vi "VisualizeRTdataExternal.vi"(0 "ExitExternalPrograms":refnum<notifier>, 2 "path":path=path "C:/Users/olaja/Dropbox (Personal)/BME/IAF DATA/March30_2021/March_30_A", 4 "RTData/PPData":bool, 5 "error in (no error)":errorcluster) -> (19 "error out":errorcluster)   [LabVIEW 2021]
uses:
  <vilib>/Utility/file.llb/Read Delimited Spreadsheet (string).vi
  <vilib>/Utility/file.llb/Read Delimited Spreadsheet (DBL).vi
  <vilib>/Analysis/NI_AALBase.lvlib
panel:
  out "Current Experiment":string
  out "XY Graph":cluster{dbl[], dbl[]}[](graph)
  in  "Histogram intervals":i32=10
  in  "Xaxis":u16(ring) items=["Left", "Top", "Right", "Bottom", "Rotation", "CenterOfMassX", "CenterOfMassY", "FirstPixelY", "Area", "Mean Intensity", "Standard  Deviation", "Minimum Intensity", "Maximum Intensity", "FrameIndex"]
  in  "Yaxis":u16(ring) items=["Left", "Top", "Right", "Bottom", "Rotation", "CenterOfMassX", "CenterOfMassY", "FirstPixelY", "Area", "Mean Intensity", "Standard  Deviation", "Minimum Intensity", "Maximum Intensity", "FrameIndex"]
  out "Histogram Graph":T1(graph)
  in  "Refresh":bool
  # "If you want to visualize a new Experiment, Close this window and open it again from Main UI"
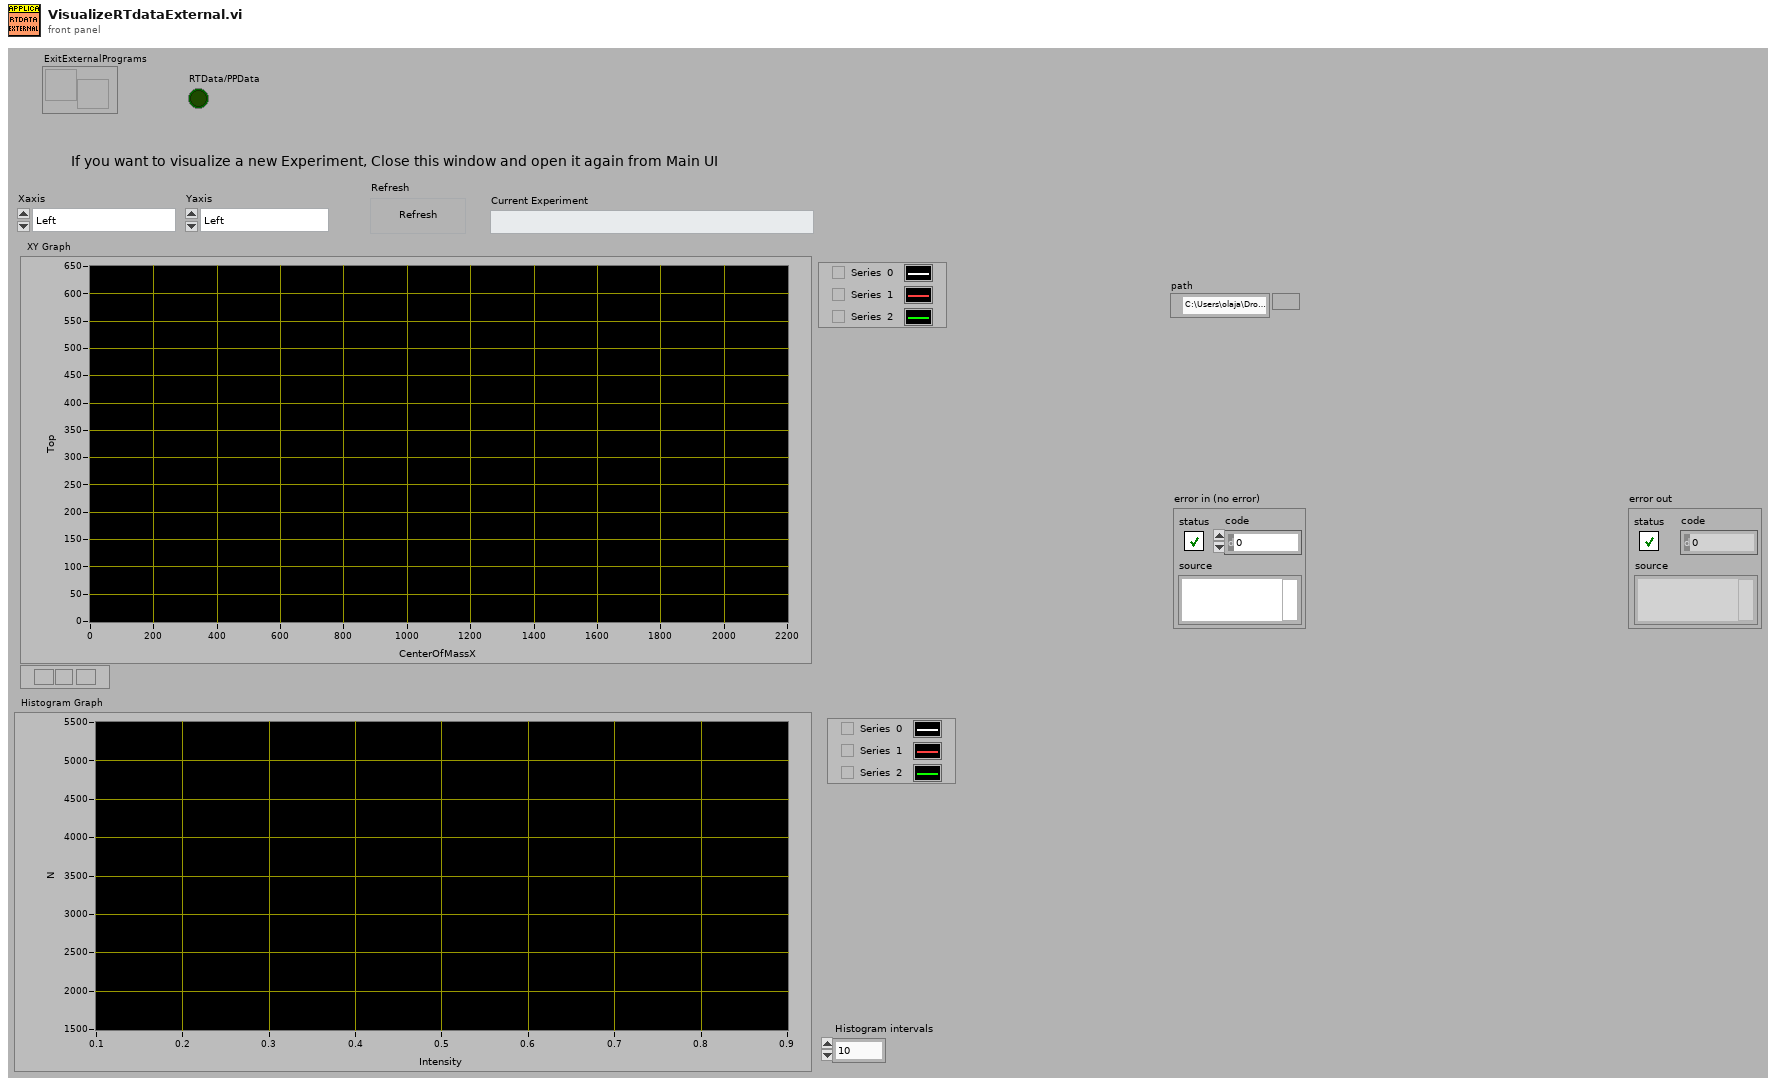
[diagram p1: front panel]
types:
  T1 = cluster{"X Values":dbl[], "Histogram: h(x)":i32[]}[]
  T2 = cluster{"X Values":dbl[], "Histogram: h(x)":i32[]}
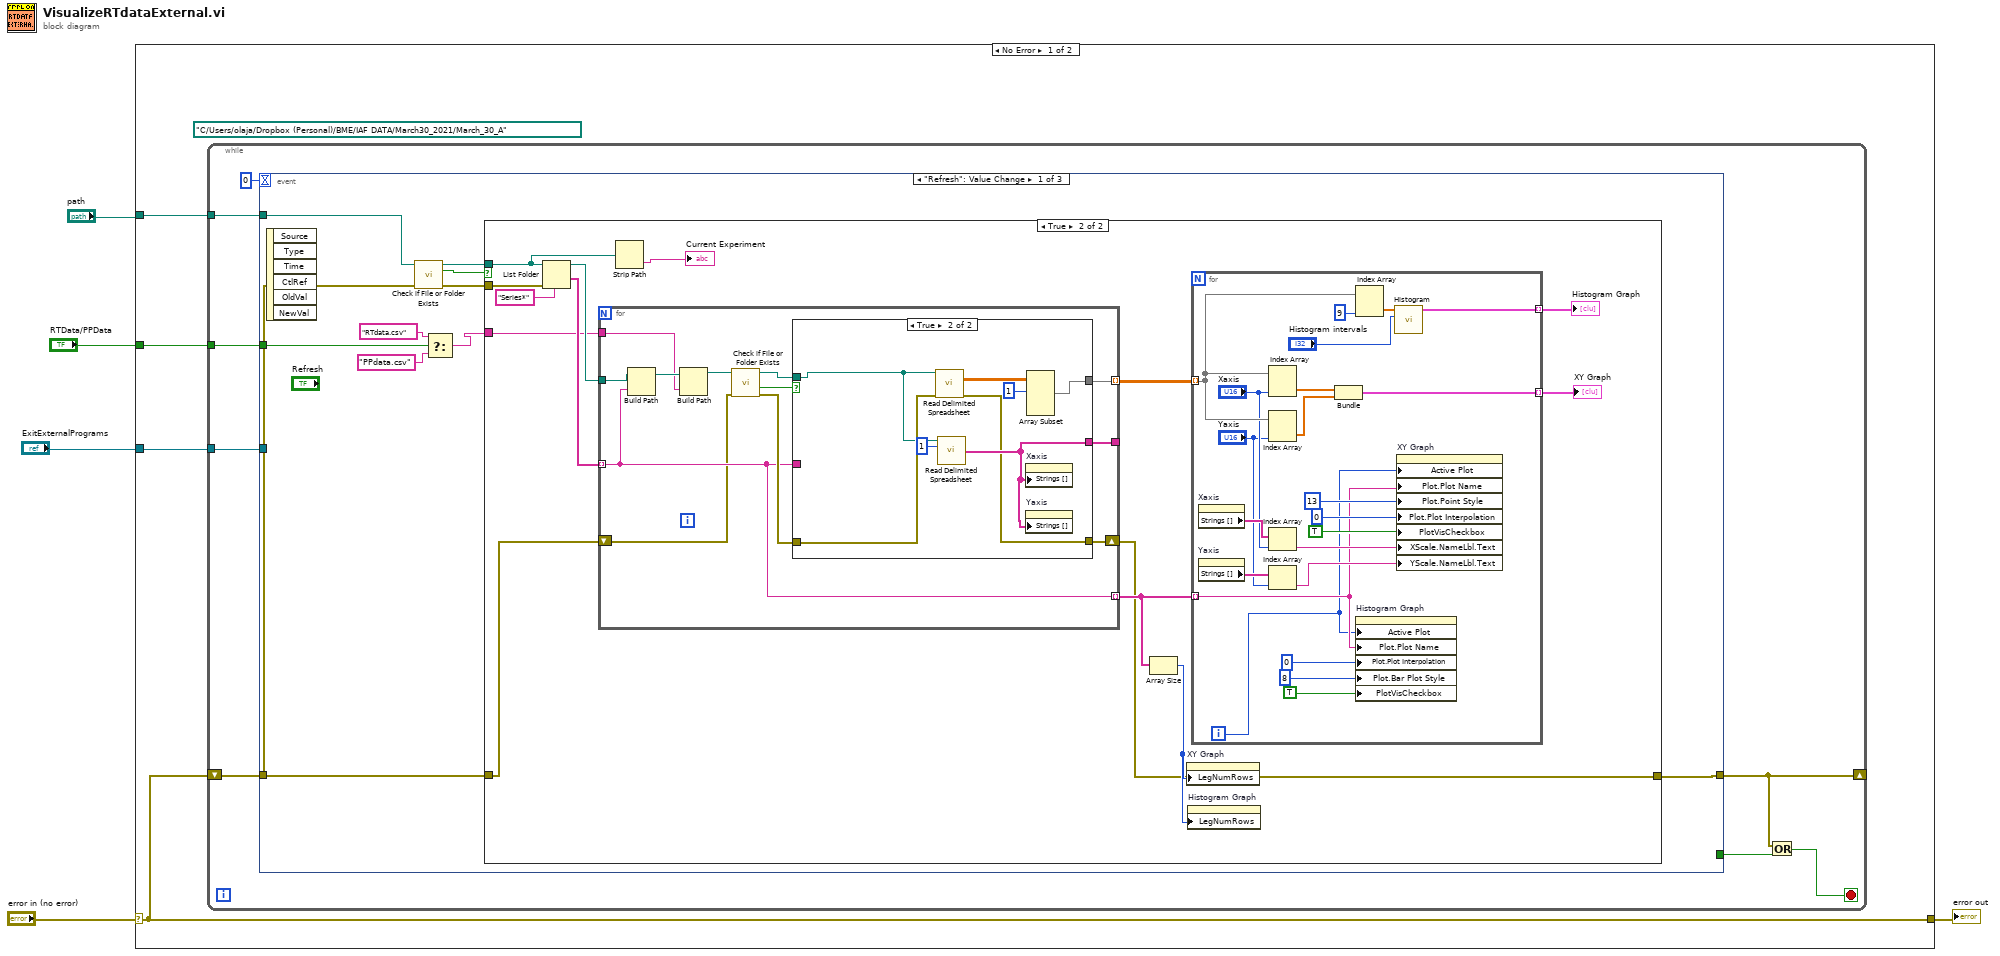
[diagram p0: block diagram]
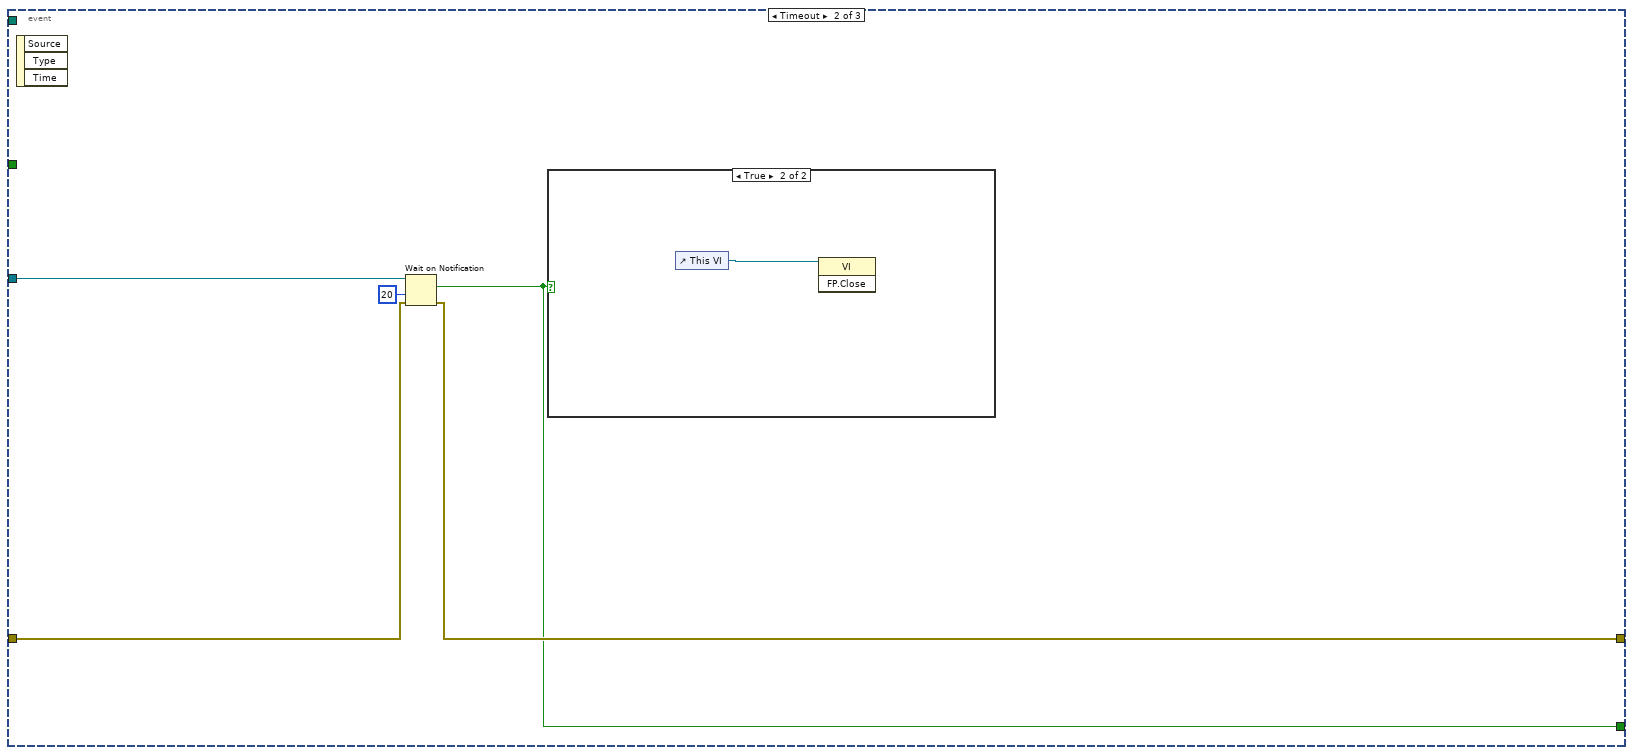
[diagram p4: hidden frame]
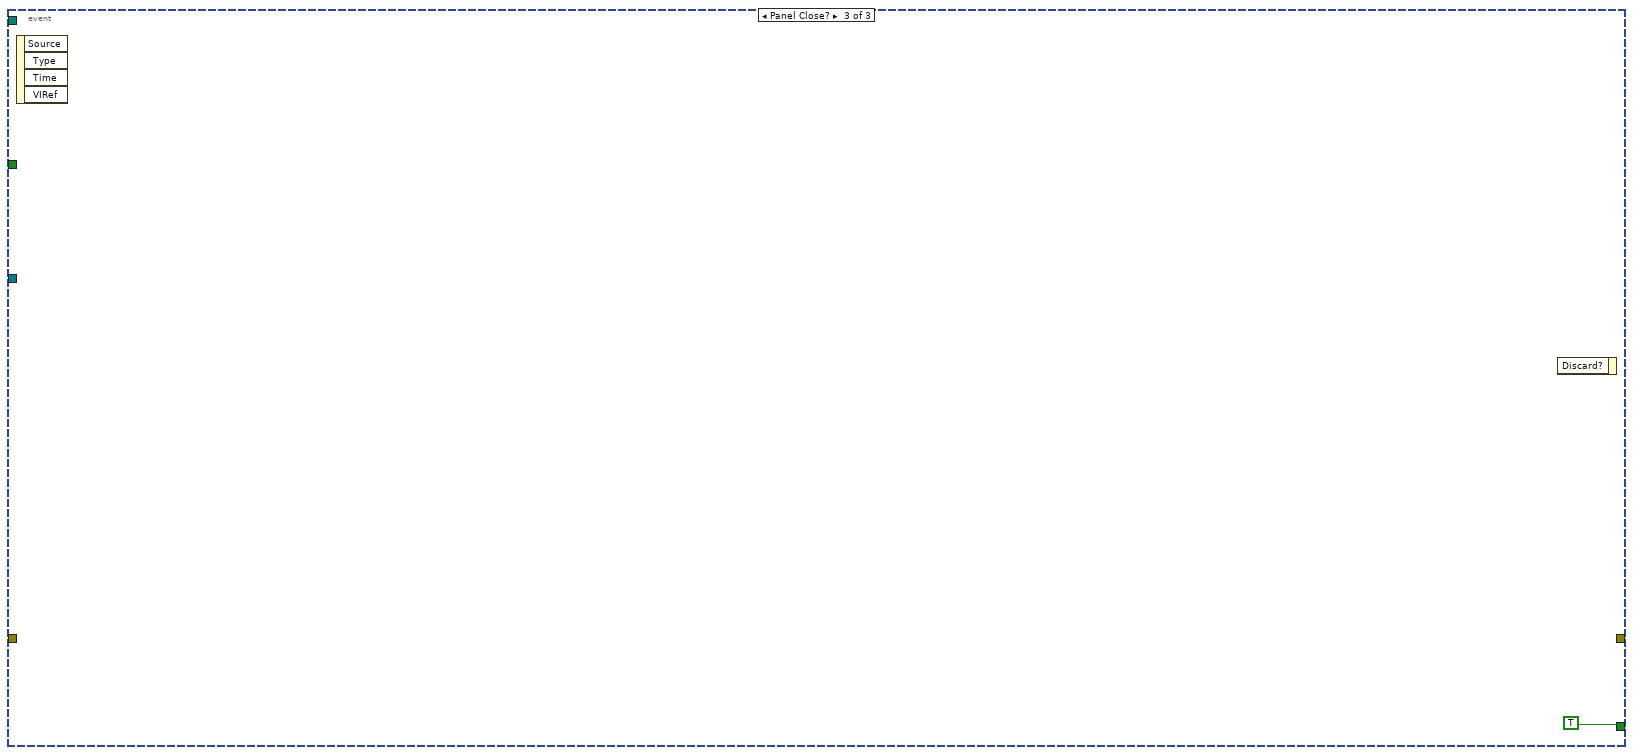
[diagram p6: hidden frame]
diagram:
  n1 = case shown="No Error" "error in (no error)" {
    selector: "error in (no error)" -> [w9 w93]
    tunnel: [w9 w93] -> w4
    tunnel: "ExitExternalPrograms" -> [w8 _]
    tunnel: "path" -> [w7 _]
    tunnel: "RTData/PPData" -> [w6 _]
    frame No Error {
      (unwired) path "C:/Users/olaja/Dropbox (Personal)/BME/IAF DATA/March30_2021/March_30_A" ("path")
      n2 = while {
        tunnel: w7 -> [w16]
        tunnel: w8 -> [w14]
        shift-right: [w13] -> _
        shift-left: w9 -> [w17]
        tunnel: w6 -> [w10]
        stop <- w11 stop-if-true
        n3 = event shown="[0] \"Refresh\": Value Change" {
          selector: _ -> [_ _ _]
          dyn-events: _ -> [_ _ _]
          timeout: 0 -> [_ _ _]
          tunnel: w17 -> [w23 w88 _]
          tunnel: [_ w86 TRUE ("Exit?")] -> w12
          tunnel: w16 -> [w24 _ _]
          tunnel: w14 -> [_ w90 _]
          tunnel: [w22 w87 _] -> w13
          tunnel: w10 -> [w18 _ _]
          event "Refresh": Value Change {
            n4 = event-data() -> ()  [unwired: 1 in, 6 out]
            n5 = call <vilib>:"Check if File or Folder Exists.vi"("error in (no error)"=w23, "path"=w24) -> ("error out"=w27:errorcluster, "file or folder exists?"=w25:bool, "dup path"=w26:path)  [unwired: 7 in]
            n6 = Select(t="RTdata.csv" ("name or relative path"), s=w18, f="PPdata.csv" ("name or relative path")) -> (s? t:f=w19:string)
            n7 = case shown="True" w25 {
              tunnel: w27 -> [_ w42]
              tunnel: w26 -> [_ w30]
              tunnel: w23 -> [w28 w33]
              tunnel: [w28 w32] -> w22
              tunnel: w19 -> [_ w31]
              frame False {
              }
              frame True {
                n8 = List Folder(path=w30, pattern="Series*", error in=w42) -> (path out=w39:path, folder names=w40:string[])  [unwired: 1 in, 2 out]
                n9 = for {
                  tunnel: w39 -> [w70]
                  tunnel: w40 -> [w68] mode=indexing
                  tunnel: [w76] -> w38 mode=indexing
                  tunnel: [w69] -> _
                  tunnel: [w68] -> w35 mode=indexing
                  shift-right: [w66] -> w32
                  shift-left: w33 -> [w67]
                  tunnel: w31 -> [w65]
                  n10 = Build Path(base path=w70, name or relative path=w68) -> (appended path=w71:path)
                  n11 = Build Path(base path=w71, name or relative path=w65) -> (appended path=w72:path)
                  n12 = call <vilib>:"Check if File or Folder Exists.vi"("error in (no error)"=w67, "path"=w72) -> ("error out"=w75:errorcluster, "file or folder exists?"=w73:bool, "dup path"=w74:path)  [unwired: 7 in]
                  n13 = case shown="True" w73 {
                    tunnel: w68 -> [_ _]
                    tunnel: [_ w79] -> w76
                    tunnel: w75 -> [w77 w85]
                    tunnel: w74 -> [_ w84]
                    tunnel: [_ w82] -> w69
                    tunnel: [w77 w78] -> w66
                    frame False {
                    }
                    frame True {
                      n14 = call-poly <vilib>:"Read Delimited Spreadsheet.vi"("file path (dialog if empty)"=w84, "error in (no error)"=w85) -> ("all rows"=w80:dbl[][], "error out"=w78:errorcluster)  [unwired: 8 in, 4 out]
                      n15 = call-poly <vilib>:"Read Delimited Spreadsheet.vi"("file path (dialog if empty)"=w84, "number of rows (all:-1)"=1) -> ("first row"=w82:string[])  [unwired: 8 in, 5 out]
                      n16 = property on="Xaxis" class="Ring (strict)"("Strings []"=w82) -> ()  [unwired: 2 in, 2 out]
                      n17 = property on="Yaxis" class="Ring (strict)"("Strings []"=w82) -> ()  [unwired: 2 in, 2 out]
                      n18 = Array Subset(array=w80, index (row)=1 ("index")) -> (w79:dbl[][])  [unwired: 3 in]
                    }
                  }
                }
                n19 = Strip Path(path=w30) -> (name=→"Current Experiment":string)  [unwired: 1 out]
                n20 = Array Size(array=w35) -> (size(s)=w34:i32)
                n21 = property on="XY Graph" class="XYGraph (strict)"("LegNumRows"=w34) -> ()  [unwired: 2 in, 2 out]
                n22 = property on="Histogram Graph" class="XYGraph (strict)"("LegNumRows"=w34) -> ()  [unwired: 2 in, 2 out]
                n23 = for {
                  tunnel: w38 -> [w58] mode=indexing
                  tunnel: [w63] -> w37 mode=indexing
                  tunnel: w35 -> [w44] mode=indexing
                  tunnel: [w59] -> w36 mode=indexing
                  i -> [w43]
                  n24 = property on="Xaxis" class="Ring (strict)"() -> ("Strings []"=w50:string[])  [unwired: 2 in, 2 out]
                  n25 = property on="Yaxis" class="Ring (strict)"() -> ("Strings []"=w47:string[])  [unwired: 2 in, 2 out]
                  n26 = Index Array(array=w58, index (col)="Xaxis") -> (element=w60:dbl[])  [unwired: 1 in]
                  n27 = Index Array(array=w58, index (col)="Yaxis") -> (element=w64:dbl[])  [unwired: 1 in]
                  n28 = Index Array(array=w50, index="Xaxis") -> (element=w48:string)
                  n29 = Index Array(array=w47, index="Yaxis") -> (element=w45:string)
                  n30 = Bundle(w60, w64) -> (w63:cluster{dbl[], dbl[]})  [unwired: 1 in]
                  n31 = Index Array(array=w58, index (col)=9 ("index (row)")) -> (element=w57:dbl[])  [unwired: 1 in]
                  n32 = property on="Histogram Graph" class="XYGraph (strict)"("Active Plot"=w43, "Plot.Plot Name"=w44, "Plot.Plot Interpolation"=u8 0, "Plot.Bar Plot Style"=u8 8, "PlotVisCheckbox"=TRUE ("Legend:Plot Visibility Checkbox Visible")) -> ()  [unwired: 2 in, 2 out]
                  n33 = call <vilib>:"Histogram.vi"("intervals"="Histogram intervals", "X"=w57) -> ("Histogram Graph"=w59:T2)  [unwired: 6 in, 3 out]
                  n34 = property on="XY Graph" class="XYGraph (strict)"("Active Plot"=w43, "Plot.Plot Name"=w44, "Plot.Point Style"=u8 13, "Plot.Plot Interpolation"=u8 0, "PlotVisCheckbox"=TRUE ("Legend:Plot Visibility Checkbox Visible"), "XScale.NameLbl.Text"=w48, "YScale.NameLbl.Text"=w45) -> ()  [unwired: 2 in, 2 out]
                }
                "XY Graph" <- w37
                "Histogram Graph" <- w36
              }
            }
          }
          event Timeout {
            n35 = event-data() -> ()  [unwired: 1 in, 3 out]
            n36 = Wait on Notification(notifier=w90, timeout in ms (-1)=20, error in (no error)=w88) -> (notification=w86:bool, error out=w87:errorcluster)  [unwired: 1 in, 2 out]
            n37 = case shown="True" w86 {
              frame False {
              }
              frame True {
                n38 = control-ref of="This VI"() -> (w91:refnum<vi>)
                n39 = invoke class="VI" method="FP.Close"(reference=w91) -> ()  [unwired: 2 in, 3 out]
              }
            }
          }
          event Panel Close? {
            n40 = event-data() -> ()  [unwired: 1 in, 4 out]
            n41 = event-data() -> ()  [unwired: 2 in, 1 out]
          }
        }
        n42 = Or(x=w13, y=w12) -> (x .or. y?=w11:bool)
      }
    }
    frame Error {
    }
  }
  "error out" <- w4
